vi "Update Pin Map.vi"(0 "pin map path":string, 2 "sequence context":refnum<k7>, 3 "error in":errorcluster) -> (10 "error out":errorcluster)   [LabVIEW 2020, in "NIFgenStandardFunction.lvlib"]
uses:
  NIFgenStandardFunction.lvlib
  <vilib>/MeasurementLink/MeasurementLink TestStand Integration/MeasurementLink TestStand Integration.lvlib
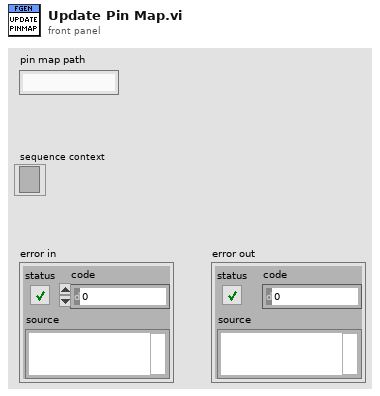
[diagram p1: front panel]
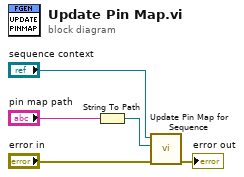
[diagram p0: block diagram]
diagram:
  n1 = String To Path(string="pin map path") -> (path=w2:path)
  n2 = call <vilib>:"Update Pin Map for Sequence.vi"("error in"="error in", "pin map path"=w2, "sequence context in"="sequence context") -> ("error out"=→"error out":errorcluster)  [unwired: 8 in]
